vi "SetOutput6 (SubVI).vi"(9 "Right":dbl, 10 "Left":dbl, 11 "DriveControlDevRef":T1) -> (3 "Motor array":dbl[](array[numeric]))   [LabVIEW 2017]
uses:
  LabVIEW Data/Skele/FRC SimulatedRSC/Motors.ctl
  <vilib>/Rock Robotics/WPI/MotorControl/WPI_MotorControlDeviceRef.ctl
  <vilib>/Rock Robotics/WPI/MotorControl/WPI_MotorControlType.ctl
  <vilib>/Rock Robotics/SystemInterfaces/DIO/FPGA_DIOPWMChannel.ctl
  <vilib>/Rock Robotics/WPI/PWM/WPI_PWMDeadband.ctl
  <vilib>/Rock Robotics/SystemInterfaces/DIO/FPGA_DIOChannel.ctl
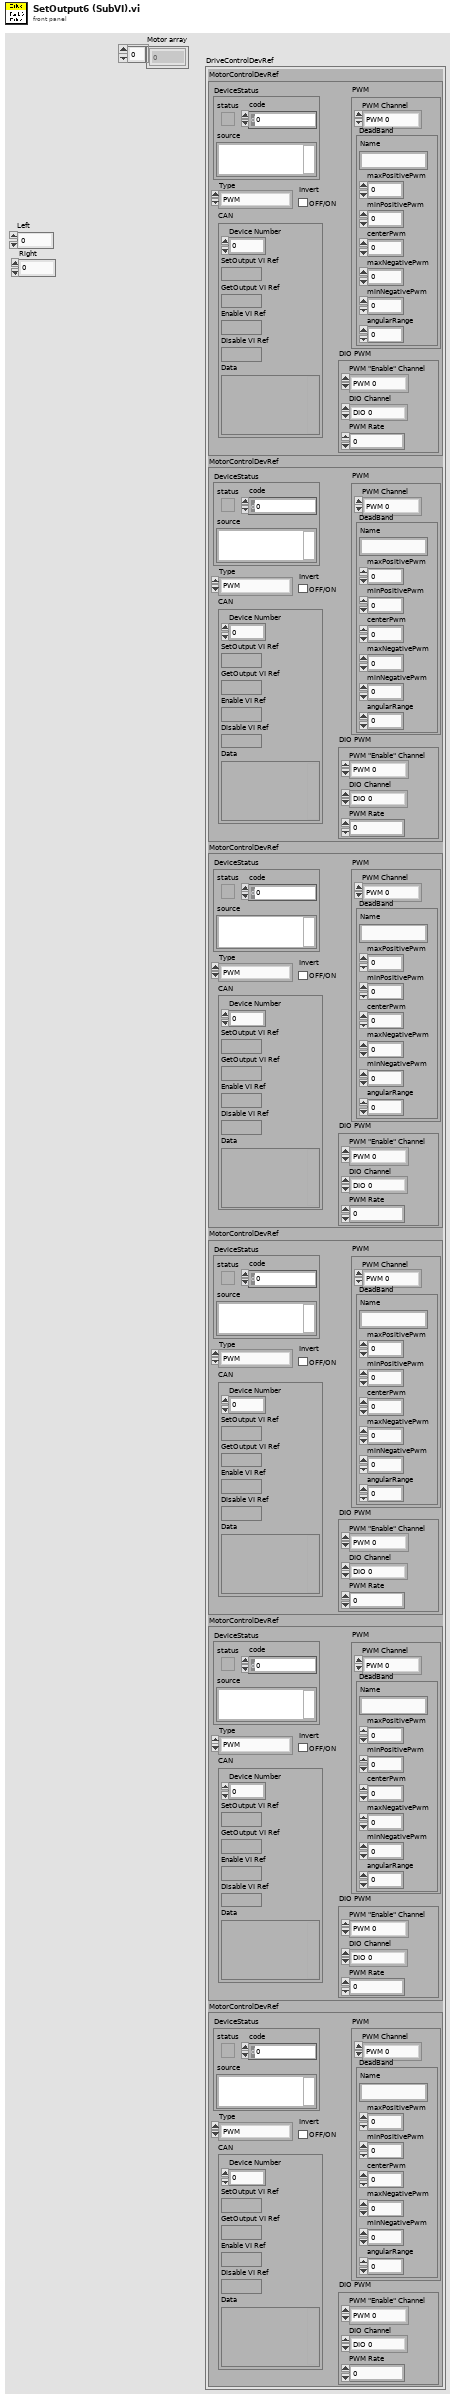
[diagram p1: front panel]
types:
  T1 = typedef "Motors.ctl" = cluster{"MotorControlDevRef":T2, "MotorControlDevRef":T2, "MotorControlDevRef":T2, "MotorControlDevRef":T2, "MotorControlDevRef":T2, "MotorControlDevRef":T2}
  T2 = typedef "WPI_MotorControlDeviceRef.ctl" = cluster{"DeviceStatus":errorcluster, "Type":T3, "PWM":cluster{"PWM Channel":T4, "DeadBand":T5}, "CAN":cluster{"Device Number":u8, "SetOutput VI Ref":variant, "GetOutput VI Ref":variant, "Enable VI Ref":variant, "Disable VI Ref":variant, "Data":variant}, "Invert":bool, "DIO PWM":cluster{"PWM \"Enable\" Channel":T4, "DIOChannel":T6, "PWM Rate":dbl}}
  T3 = typedef "WPI_MotorControlType.ctl" = enum16{"PWM", "CAN", "DIO PWM"}
  T4 = typedef "FPGA_DIOPWMChannel.ctl" = enum8{"PWM 0", "PWM 1", "PWM 2", "PWM 3", "PWM 4", "PWM 5", "PWM 6", "PWM 7", "PWM 8", "PWM 9", "PWM MXP 0", "PWM MXP 1", "PWM MXP 2", "PWM MXP 3", "PWM MXP 4", "PWM MXP 5", "PWM MXP 6", "PWM MXP 7", "PWM MXP 8", "PWM MXP 9", "Invalid"}
  T5 = typedef "WPI_PWMDeadband.ctl" = cluster{"Name":string, "maxPositivePwm":i32, "minPositivePwm":i32, "centerPwm":i32, "maxNegativePwm":i32, "minNegativePwm":i32, "angularRange":u16}
  T6 = typedef "FPGA_DIOChannel.ctl" = enum8{"DIO 0", "DIO 1", "DIO 2", "DIO 3", "DIO 4", "DIO 5", "DIO 6", "DIO 7", "DIO 8", "DIO 9", "DIO MXP 0", "DIO MXP 1", "DIO MXP 2", "DIO MXP 3", "DIO MXP 4", "DIO MXP 5", "DIO MXP 6", "DIO MXP 7", "DIO MXP 8", "DIO MXP 9", "DIO MXP 10", "DIO MXP 11", "DIO MXP 12", "DIO MXP 13", "DIO MXP 14", "DIO MXP 15", "SPI Port CS1", "SPI Port CS2", "SPI Port CS3", "SPI Port MISO", "SPI Port MOSI", "Invalid"}
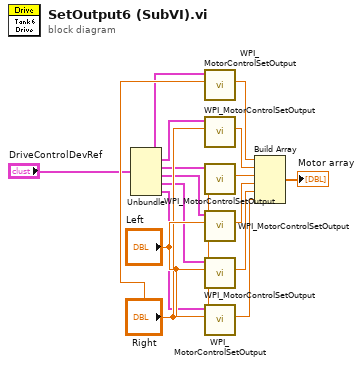
[diagram p0: block diagram]
diagram:
  n1 = Unbundle("DriveControlDevRef") -> ("MotorControlDevRef"=w13:T2, "MotorControlDevRef"=w12:T2, "MotorControlDevRef"=w11:T2, "MotorControlDevRef"=w10:T2, "MotorControlDevRef"=w9:T2, "MotorControlDevRef"=w8:T2)
  n2 = call <vilib>:"WPI_MotorControlSetOutput.vi"("Output"="Right", "MotorControlDevRef"=w13) -> ("Motor Output"=w7:dbl)  [unwired: 7 in, 2 out]
  n3 = call <vilib>:"WPI_MotorControlSetOutput.vi"("Output"="Right", "MotorControlDevRef"=w12) -> ("Motor Output"=w6:dbl)  [unwired: 7 in, 2 out]
  n4 = call <vilib>:"WPI_MotorControlSetOutput.vi"("Output"="Right", "MotorControlDevRef"=w11) -> ("Motor Output"=w5:dbl)  [unwired: 7 in, 2 out]
  n5 = call <vilib>:"WPI_MotorControlSetOutput.vi"("Output"="Left", "MotorControlDevRef"=w10) -> ("Motor Output"=w4:dbl)  [unwired: 7 in, 2 out]
  n6 = call <vilib>:"WPI_MotorControlSetOutput.vi"("Output"="Left", "MotorControlDevRef"=w9) -> ("Motor Output"=w3:dbl)  [unwired: 7 in, 2 out]
  n7 = call <vilib>:"WPI_MotorControlSetOutput.vi"("Output"="Left", "MotorControlDevRef"=w8) -> ("Motor Output"=w2:dbl)  [unwired: 7 in, 2 out]
  n8 = Build Array(w7, w6, w5, w4, w3, w2) -> (→"Motor array":dbl[])
